vi "TCP-KO-Send Command.vi"(0 "connection ID":refnum<k5>, 7 "Command":string, 9 "timeout (ms)":i32=5000, 11 "error in (no error)":errorcluster, 12 "fast response":bool) -> (4 "connection ID out":refnum<k5>, 15 "error out":errorcluster)   [LabVIEW 2020]
panel:
  out "result":i32
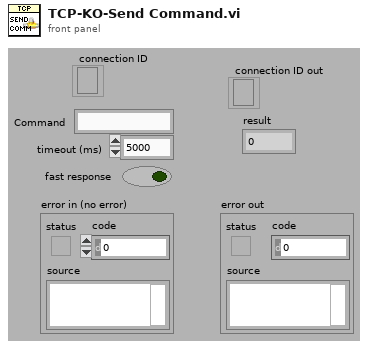
[diagram p1: front panel]
types:
  T1 = enum16{"Standard", "Buffered", "CRLF", "Immediate"}
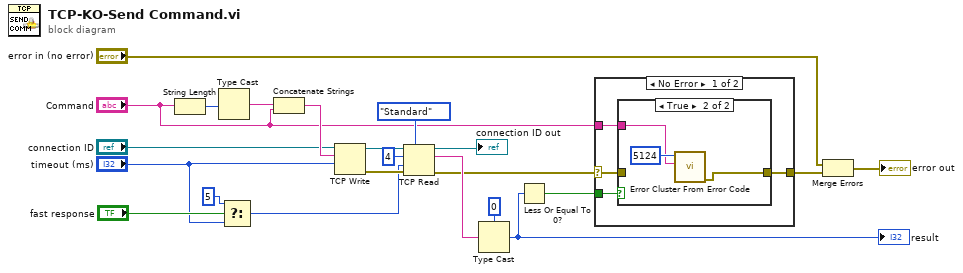
[diagram p0: block diagram]
diagram:
  n1 = String Length(string="Command") -> (length=w21:i32)
  n2 = Type Cast(x=w21) -> (*(type *) &x=w20:string)  [unwired: 1 in]
  n3 = Select(t=5 ("timeout ms (25000)"), s="fast response", f="timeout (ms)") -> (s? t:f=w6:i32)
  n4 = Concatenate Strings(w20, "Command") -> (w22:string)
  n5 = TCP Write(connection ID="connection ID", data in=w22, 9:"timeout (ms)") -> (connection ID out=w19:refnum<k5>, error out=w10:errorcluster)  [unwired: 1 in, 1 out]
  n6 = TCP Read(connection ID=w19, bytes to read=4, error in (no error)=w10, 7:T1."Standard" ("mode (standard)"), 9:w6) -> (connection ID out=→"connection ID out":refnum<k5>, data out=w18:string, error out=w9:errorcluster)
  n7 = Type Cast(type=0, x=w18) -> (*(type *) &x=w4:i32)
  "result" <- w4
  n8 = Less Or Equal To 0?(x=w4) -> (x <= 0?=w16:bool)
  n9 = case shown="No Error" w9 {
    selector: w9 -> [w24 w31]
    tunnel: w16 -> [w26 _]
    tunnel: [w25 w31] -> w15
    tunnel: "Command" -> [w23 _]
    frame No Error {
      n10 = case shown="True" w26 {
        tunnel: [w27 w28] -> w25
        tunnel: w24 -> [w27 _]
        tunnel: w23 -> [_ w29]
        frame False {
        }
        frame True {
          n11 = call <vilib>:"Error Cluster From Error Code.vi"("error message (\"\")"=w29, "error code (0)"=5124) -> ("error out"=w28:errorcluster)  [unwired: 7 in]
        }
      }
    }
    frame Error {
    }
  }
  n12 = Merge Errors("error in (no error)", w15) -> (→"error out":errorcluster)
